vi "产品高低配.vi"(1 "低配":bool, 2 "高配":bool) -> (0 "产品高低配":i16)   [LabVIEW 2018]
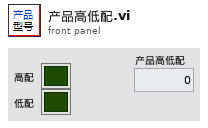
[diagram p1: front panel]
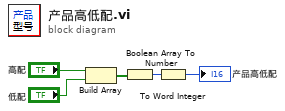
[diagram p0: block diagram]
diagram:
  n1 = Build Array("高配", "低配") -> (w3:bool[])
  n2 = Boolean Array To Number(Boolean array=w3) -> (number=w2:u32)
  n3 = To Word Integer(number=w2) -> (16bit integer=→"产品高低配":i16)
